vi "InsertBinData.vi"(8 "error in (no error)":errorcluster, 9 "FileName":string, 10 "string":string, 11 "connection reference":T1) -> (0 "error out":errorcluster, 1 "concatenated string":string, 3 "connection reference out":T1)   [LabVIEW 2012]
uses:
  <vilib>/addons/database/Connection.llb/Conn ObjectReference.ctl
  <vilib>/addons/database/NI_Database_API.lvlib
panel:
  out "after substring":string
  in  "input cluster":T2
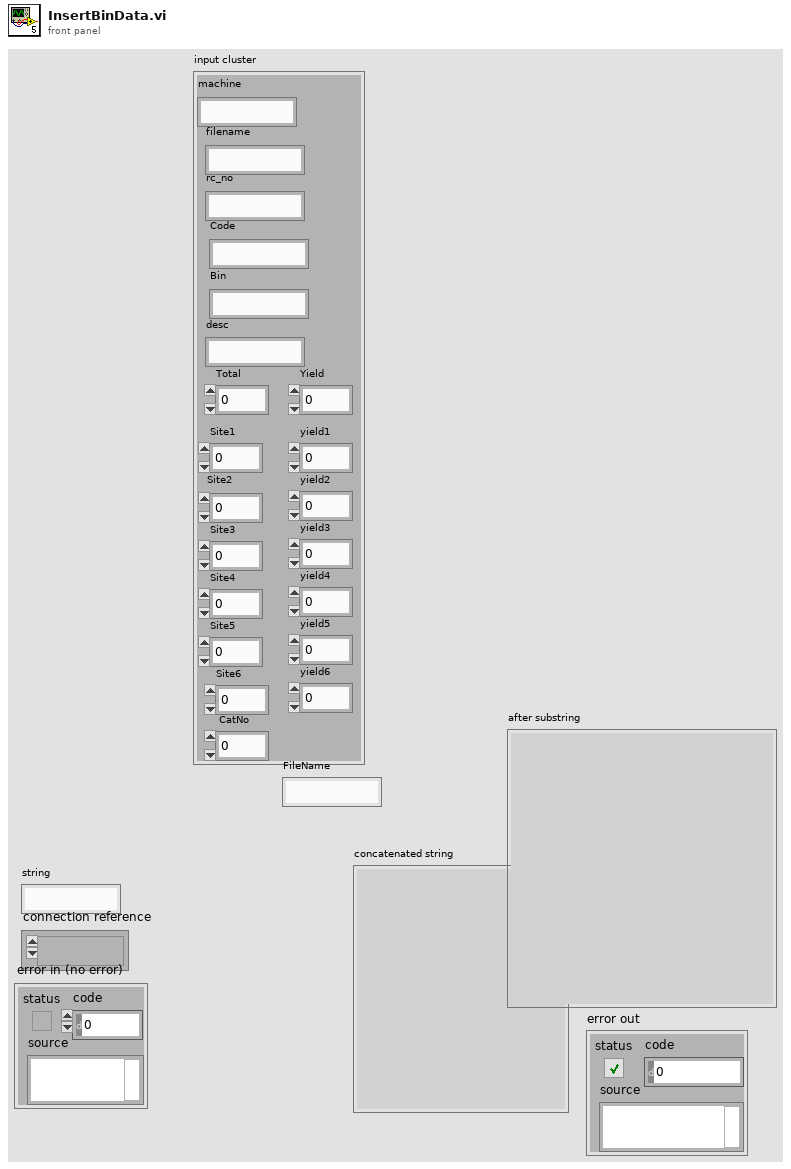
[diagram p1: front panel]
types:
  T1 = typedef "NI_Database_API.lvlib/Conn ObjectReference.ctl" = refnum<k1>
  T2 = cluster{"machine":string, "filename":string, "rc_no":string, "Code":string, "Bin":string, "desc":string, "Total":dbl, "Yield":dbl, "Site1":dbl, "yield1":dbl, "Site2":dbl, "yield2":dbl, "Site3":dbl, "yield3":dbl, "Site4":dbl, "yield4":dbl, "Site5":dbl, "yield5":dbl, "Site6":dbl, "yield6":dbl, " CatNo":dbl}
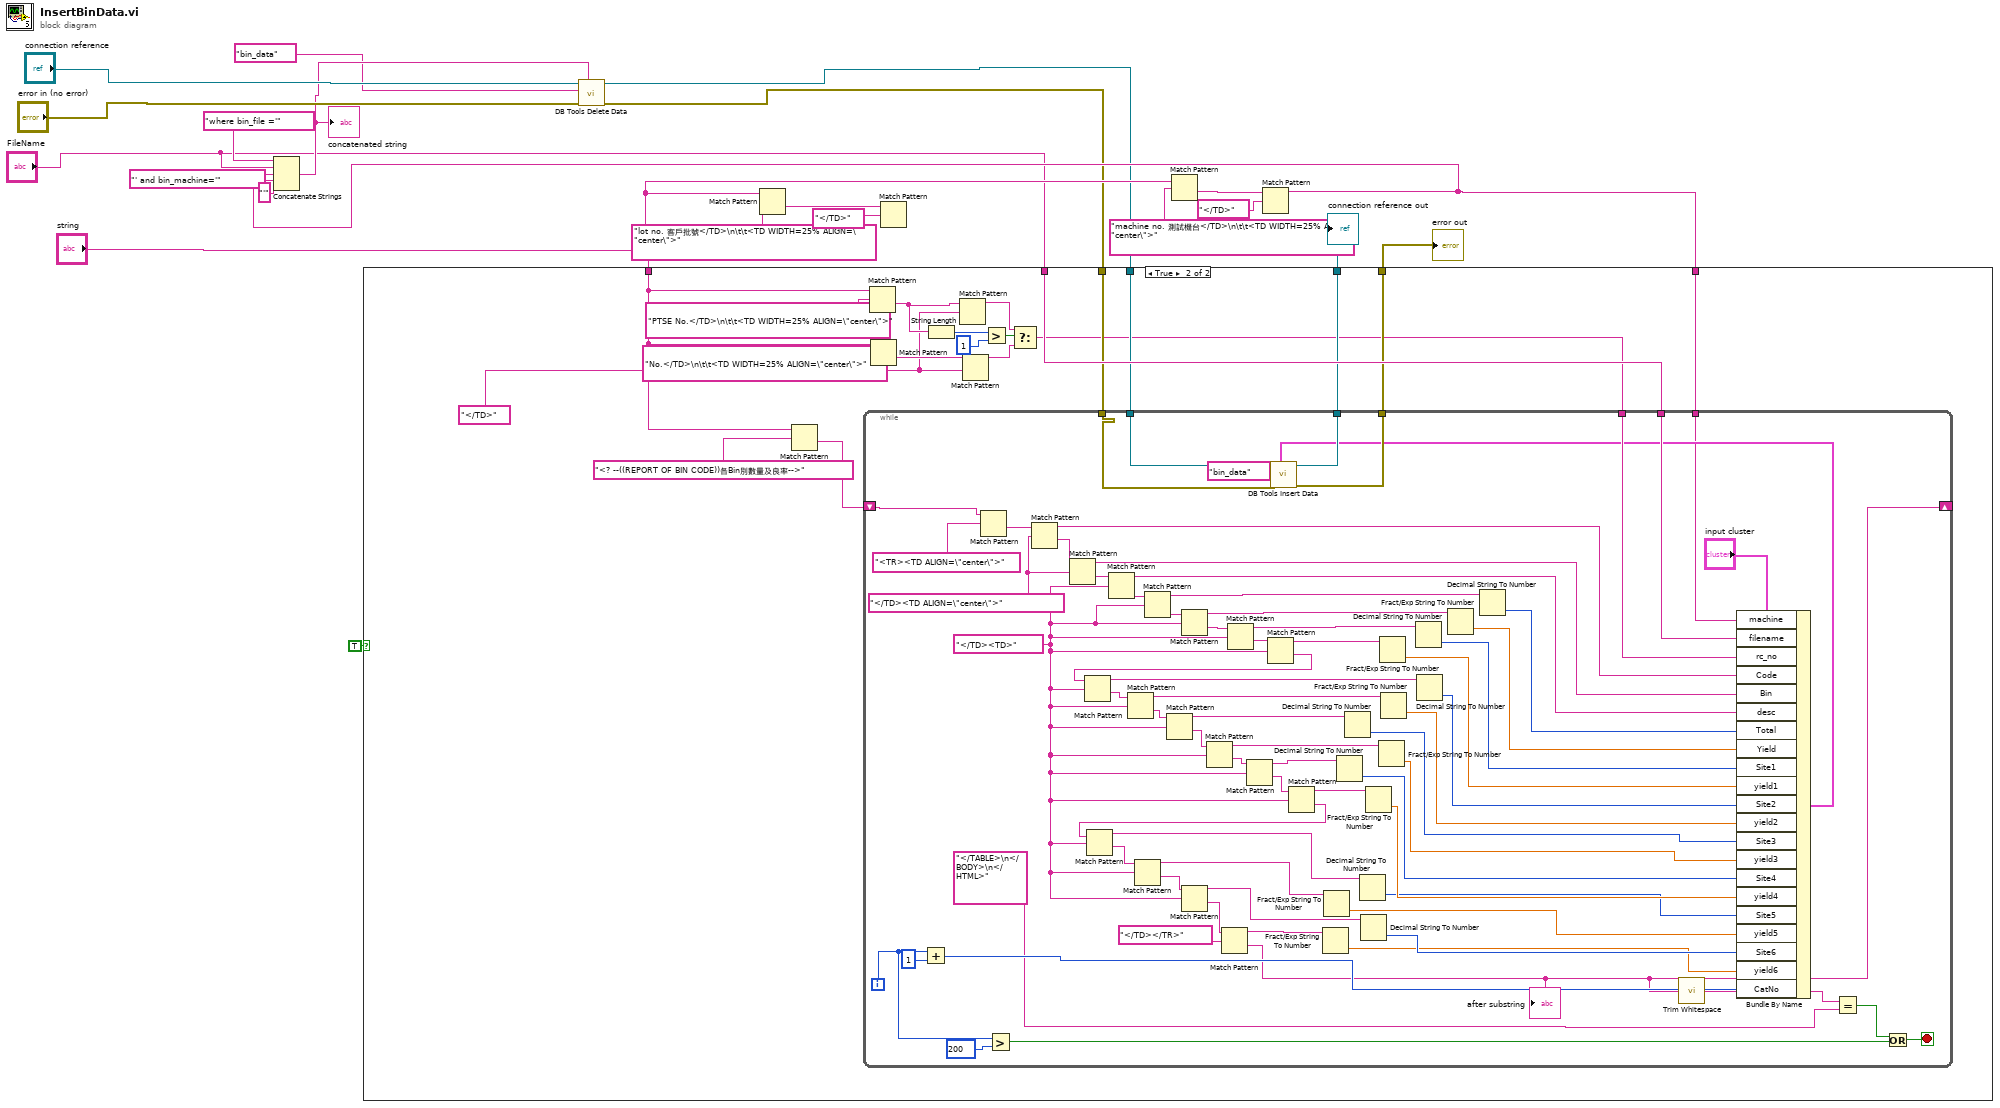
[diagram p0: block diagram]
diagram:
  n1 = Match Pattern(string="string", regular expression="lot no. 客戶批號</TD>\n\t\t<TD WIDTH=25% ALIGN=\"center\">") -> (after substring=w18:string)  [unwired: 1 in, 3 out]
  n2 = Match Pattern(string=w18, regular expression="</TD>") -> ()  [unwired: 1 in, 4 out]
  n3 = Match Pattern(string="string", regular expression="machine no. 測試機台</TD>\n\t\t<TD WIDTH=25% ALIGN=\"center\">") -> (after substring=w10:string)  [unwired: 1 in, 3 out]
  n4 = Match Pattern(string=w10, regular expression="</TD>") -> (before substring=w7:string)  [unwired: 1 in, 3 out]
  n5 = Concatenate Strings("where bin_file ='" ("SQL query"), "FileName", "' and bin_machine='" ("string"), w7, "'" ("string")) -> (w5:string)
  "concatenated string" <- w5
  n6 = call <vilib>:"DB Tools Delete Data.vi"("condition"=w5, "error in (no error)"="error in (no error)", "table"="bin_data", "connection reference"="connection reference") -> ("error out"=w2:errorcluster, "connection reference out"=w3:T1)  [unwired: 6 in]
  n7 = case shown="True" TRUE {
    tunnel: "string" -> [_ w26]
    tunnel: "FileName" -> [_ w32]
    tunnel: w3 -> [w23 w31]
    tunnel: [w23 w30] -> w21
    tunnel: [w22 w29] -> w20
    tunnel: w2 -> [w22 w28]
    tunnel: w7 -> [_ w27]
    frame False {
    }
    frame True {
      w25 = "</TD>" ("regular expression")
      n8 = Match Pattern(string=w26, regular expression="<? --((REPORT OF BIN CODE))各Bin別數量及良率-->") -> (after substring=w33:string)  [unwired: 1 in, 3 out]
      n9 = Match Pattern(string=w26, regular expression="PTSE No.</TD>\n\t\t<TD WIDTH=25% ALIGN=\"center\">") -> (after substring=w40:string)  [unwired: 1 in, 3 out]
      n10 = Match Pattern(string=w26, regular expression="No.</TD>\n\t\t<TD WIDTH=25% ALIGN=\"center\">") -> (after substring=w42:string)  [unwired: 1 in, 3 out]
      n11 = String Length(string=w40) -> (length=w38:i32)
      n12 = Match Pattern(string=w40, regular expression=w25) -> (before substring=w36:string)  [unwired: 1 in, 3 out]
      n13 = Match Pattern(string=w42, regular expression=w25) -> (before substring=w35:string)  [unwired: 1 in, 3 out]
      n14 = Greater?(x=w38, y=1) -> (0:w39:bool)
      n15 = Select(t=w36, s=w39, f=w35) -> (s? t:f=w24:string)
      n16 = while {
        shift-right: [w50] -> _
        shift-left: w33 -> [w96]
        tunnel: w32 -> [w93]
        tunnel: w24 -> [w92]
        tunnel: w31 -> [w59]
        tunnel: [w58] -> w30
        tunnel: [w57] -> w29
        tunnel: w28 -> [w55]
        tunnel: w27 -> [w54]
        i -> [w46]
        stop <- w48 stop-if-true
        w97 = "</TD><TD>" ("regular expression")
        w112 = "</TD><TD ALIGN=\"center\">" ("regular expression")
        n17 = Add(x=w46, y=1) -> (x+y=w52:i32)
        n18 = Match Pattern(string=w96, regular expression="<TR><TD ALIGN=\"center\">") -> (after substring=w115:string)  [unwired: 1 in, 3 out]
        n19 = Greater?(x=w46, y=200) -> (0:w44:bool)
        n20 = Match Pattern(string=w115, regular expression=w112) -> (before substring=w91:string, after substring=w114:string)  [unwired: 1 in, 2 out]
        n21 = Match Pattern(string=w114, regular expression=w112) -> (before substring=w90:string, after substring=w113:string)  [unwired: 1 in, 2 out]
        n22 = Match Pattern(string=w113, regular expression=w97) -> (before substring=w89:string, after substring=w111:string)  [unwired: 1 in, 2 out]
        n23 = Match Pattern(string=w111, regular expression=w97) -> (before substring=w87:string, after substring=w110:string)  [unwired: 1 in, 2 out]
        n24 = Match Pattern(string=w110, regular expression=w97) -> (before substring=w86:string, after substring=w109:string)  [unwired: 1 in, 2 out]
        n25 = Match Pattern(string=w109, regular expression=w97) -> (before substring=w85:string, after substring=w108:string)  [unwired: 1 in, 2 out]
        n26 = Match Pattern(string=w108, regular expression=w97) -> (before substring=w81:string, after substring=w107:string)  [unwired: 1 in, 2 out]
        n27 = Match Pattern(string=w107, regular expression=w97) -> (before substring=w79:string, after substring=w106:string)  [unwired: 1 in, 2 out]
        n28 = Match Pattern(string=w106, regular expression=w97) -> (before substring=w78:string, after substring=w105:string)  [unwired: 1 in, 2 out]
        n29 = Match Pattern(string=w105, regular expression=w97) -> (before substring=w76:string, after substring=w104:string)  [unwired: 1 in, 2 out]
        n30 = Match Pattern(string=w104, regular expression=w97) -> (before substring=w74:string, after substring=w103:string)  [unwired: 1 in, 2 out]
        n31 = Match Pattern(string=w103, regular expression=w97) -> (before substring=w71:string, after substring=w102:string)  [unwired: 1 in, 2 out]
        n32 = Match Pattern(string=w102, regular expression=w97) -> (before substring=w69:string, after substring=w98:string)  [unwired: 1 in, 2 out]
        n33 = Match Pattern(string=w98, regular expression=w97) -> (before substring=w67:string, after substring=w101:string)  [unwired: 1 in, 2 out]
        n34 = Match Pattern(string=w101, regular expression=w97) -> (before substring=w63:string, after substring=w100:string)  [unwired: 1 in, 2 out]
        n35 = Match Pattern(string=w100, regular expression=w97) -> (before substring=w62:string, after substring=w99:string)  [unwired: 1 in, 2 out]
        n36 = Match Pattern(string=w99, regular expression="</TD></TR>") -> (before substring=w61:string, after substring=w50:string)  [unwired: 1 in, 2 out]
        "after substring" <- w50
        n37 = Fract/Exp String To Number(string=w61) -> (number=w64:dbl)  [unwired: 3 in, 1 out]
        n38 = Fract/Exp String To Number(string=w63) -> (number=w66:dbl)  [unwired: 3 in, 1 out]
        n39 = Decimal String To Number(string=w71) -> (number=w73:i32)  [unwired: 2 in, 1 out]
        n40 = Decimal String To Number(string=w76) -> (number=w75:i32)  [unwired: 2 in, 1 out]
        n41 = Decimal String To Number(string=w67) -> (number=w68:i32)  [unwired: 2 in, 1 out]
        n42 = Decimal String To Number(string=w62) -> (number=w65:i32)  [unwired: 2 in, 1 out]
        n43 = Fract/Exp String To Number(string=w69) -> (number=w70:dbl)  [unwired: 3 in, 1 out]
        n44 = Fract/Exp String To Number(string=w74) -> (number=w72:dbl)  [unwired: 3 in, 1 out]
        n45 = Fract/Exp String To Number(string=w81) -> (number=w82:dbl)  [unwired: 3 in, 1 out]
        n46 = Fract/Exp String To Number(string=w78) -> (number=w77:dbl)  [unwired: 3 in, 1 out]
        n47 = Decimal String To Number(string=w85) -> (number=w83:i32)  [unwired: 2 in, 1 out]
        n48 = Decimal String To Number(string=w79) -> (number=w80:i32)  [unwired: 2 in, 1 out]
        n49 = Fract/Exp String To Number(string=w86) -> (number=w84:dbl)  [unwired: 3 in, 1 out]
        n50 = Decimal String To Number(string=w87) -> (number=w88:i32)  [unwired: 2 in, 1 out]
        n51 = call <vilib>:"Trim Whitespace.vi"("string"=w50) -> ("trimmed string"=w49:string)  [unwired: 1 in]
        n52 = Bundle By Name(cluster="input cluster", "machine"=w54, "filename"=w93, "rc_no"=w92, "Code"=w91, "Bin"=w90, "desc"=w89, "Total"=w88, "Yield"=w84, "Site1"=w83, "yield1"=w82, "Site2"=w80, "yield2"=w77, "Site3"=w75, "yield3"=w72, "Site4"=w73, "yield4"=w70, "Site5"=w68, "yield5"=w66, "Site6"=w65, "yield6"=w64, "CatNo"=w52) -> (w56:T2)
        n53 = call <vilib>:"DB Tools Insert Data.vi"("data"=w56, "error in (no error)"=w55, "table"="bin_data", "connection reference"=w59) -> ("error out"=w57:errorcluster, "connection reference out"=w58:T1)  [unwired: 6 in]
        n54 = Equal?(x=w49, y="</TABLE>\n</BODY>\n</HTML>") -> (x = y?=w47:bool)
        n55 = Or(x=w47, y=w44) -> (x .or. y?=w48:bool)
      }
    }
  }
  "connection reference out" <- w21
  "error out" <- w20
